vi "Init Runtime.vi"(8 "error in (no error)":errorcluster, 11 "Report Config in":refnum<class "Report Config.lvclass">) -> (0 "error out":errorcluster, 2 "Report.lvclass":refnum<class "Report.lvclass">, 3 "Report Config out":refnum<class "Report Config.lvclass">)   [LabVIEW 2015, in "Report Config.lvclass"]
doc: "This VI returns a runtime class for the Report using the configuration provided."
uses:
  Report Config.lvclass
  Execution/Report.lvclass
  Report Config.lvclass/Report Config.ctl
  Report Formatters/Base Class/Config/Formatter Config.lvclass
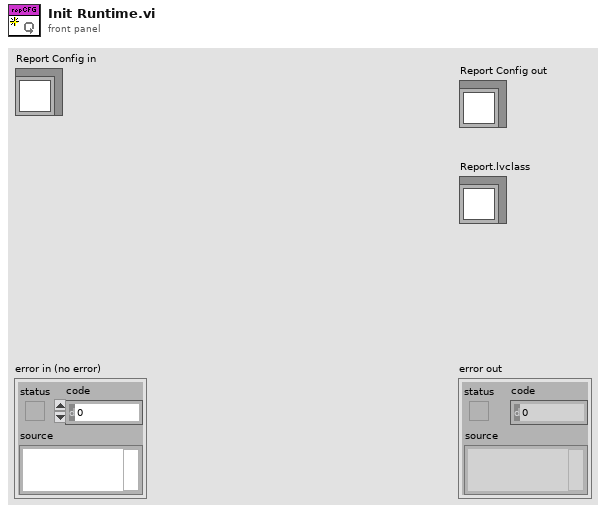
[diagram p1: front panel]
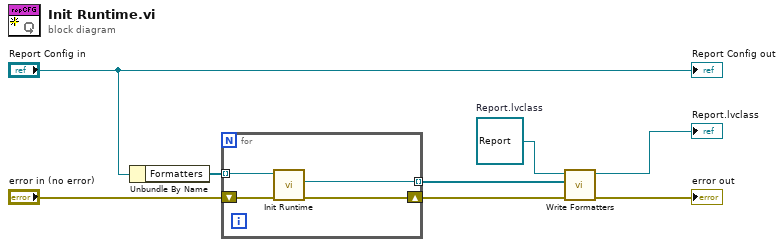
[diagram p0: block diagram]
diagram:
  w8 = refnum<class "Report.lvclass"> refnum  # Report.lvclass
  n1 = Unbundle By Name("Report Config in") -> ("Formatters"=w5:refnum<class "Formatter Config.lvclass">[])
  n2 = for {
    tunnel: w5 -> [w12] mode=indexing
    tunnel: [w11] -> w4 mode=indexing
    shift-right: [w9] -> w3
    shift-left: "error in (no error)" -> [w10]
    n3 = call-dynamic "Init Runtime.vi"("error in (no error)"=w10, "Formatter Config in"=w12) -> ("error out"=w9:errorcluster, "Formatter.lvclass"=w11:refnum<class "Formatter.lvclass">)  [unwired: 7 in, 1 out]
  }
  n4 = call-dynamic "Write Formatters.vi"("error in (no error)"=w3, "Formatters"=w4, "Report in"=w8) -> ("error out"=→"error out":errorcluster, "Report out"=→"Report.lvclass":refnum<class "Report.lvclass">)  [unwired: 7 in]
  "Report Config out" <- "Report Config in"
